vi "Teleop.vi"(6 "Intake speed axis":dbl, 8 "Auto Center":bool, 9 "Outtake":bool, 10 "Intake":bool, 11 "intake.lvclass":refnum<class "intake.lvclass">) -> (2 "State":T1, 3 "intake.lvclass":refnum<class "intake.lvclass">)   [LabVIEW 2015, in "intake.lvclass"]
uses:
  intake.lvclass
  Intake States.ctl
  Robot Global Data.vi
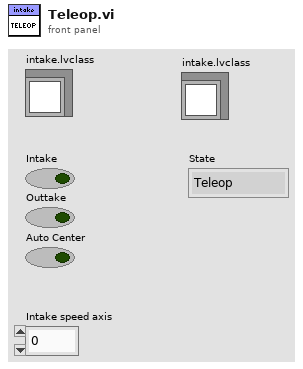
[diagram p1: front panel]
types:
  T1 = typedef "Intake States.ctl" = enum16{"Teleop", "Centering In", "Centering Out"}
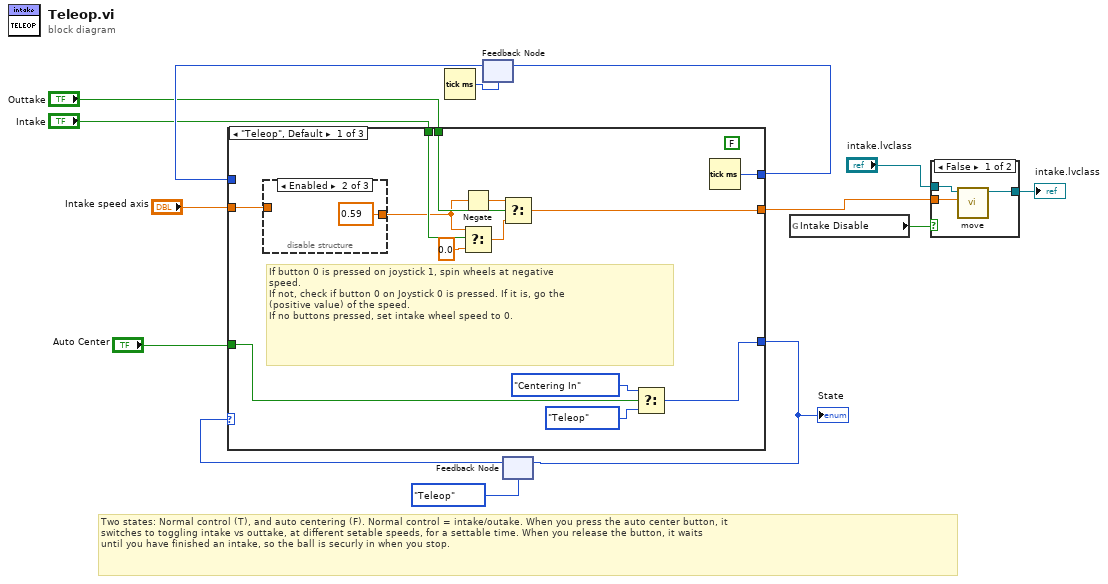
[diagram p0: block diagram]
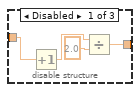
[diagram p2: hidden frame]
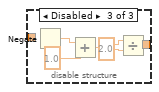
[diagram p3: hidden frame]
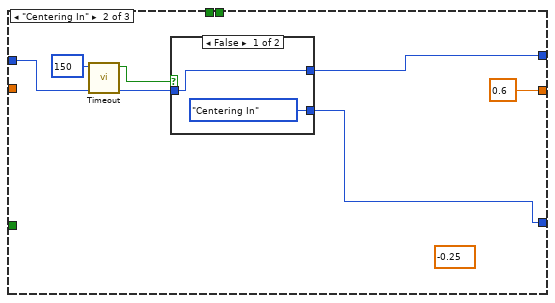
[diagram p4: hidden frame]
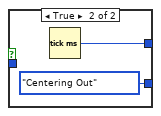
[diagram p5: hidden frame]
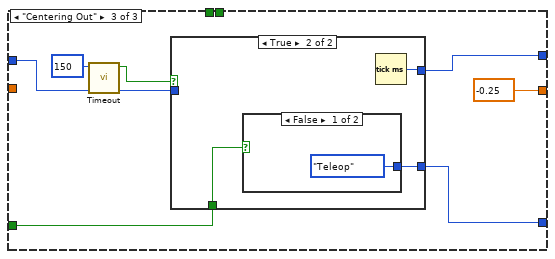
[diagram p6: hidden frame]
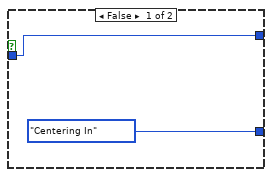
[diagram p7: hidden frame]
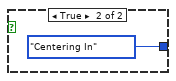
[diagram p8: hidden frame]
diagram:
  # "Two states: Normal control (T), and auto centering (F). Normal control = intake/outake. When you press the auto center button, it \nswitches to toggling intake vs outtake, at different setable speeds, for a settable time. When you release the button, it waits\nuntil you have finished an intake, so the ball is securly in when you stop."
  n1 = Tick Count (ms)() -> (millisecond timer value=w10:u32)
  n2 = feedback #1(w10) -> (w11:u32)
  n3 = feedback #2(Intake_States."Teleop" ("Enum")) -> (w1:T1)
  n4 = case shown="\"Teleop\", Default" w1 {
    tunnel: "Outtake" -> [w25 _ _]
    tunnel: "Intake" -> [w24 _ _]
    tunnel: "Intake speed axis" -> [w22 _ _]
    tunnel: [w20 0.6 ("t") -0.25 ("f")] -> w13
    tunnel: [w19 w41 w53] -> w12
    tunnel: w11 -> [_ w43 w55]
    tunnel: [w15 w38 w51] -> w9
    tunnel: "Auto Center" -> [w18 _ w49]
    frame "Teleop", Default {
      (unwired) FALSE ("Intake Disable")
      # "If button 0 is pressed on joystick 1, spin wheels at negative\nspeed.\nIf not, check if button 0 on Joystick 0 is pressed. If it is, go the\n(positive value) of the speed.\nIf no buttons pressed, set intake wheel speed to 0."
      n5 = disable-structure shown="Enabled" {
        disable-tunnel: w22 -> [w31 _ _]
        disable-tunnel: [w28 0.59 w36] -> w21
        frame Disabled {
          n6 = Increment(x=w31) -> (x+1=w30:dbl)
          n7 = Divide(x=w30, y=2.0) -> (x/y=w28:dbl)
        }
        frame Enabled {
        }
        frame Disabled {
          n8 = Negate() -> (-x=w35:dbl)  [unwired: 1 in]
          n9 = Add(x=w35, y=1.0) -> (x+y=w33:dbl)
          n10 = Divide(x=w33, y=2.0) -> (x/y=w36:dbl)
        }
      }
      n11 = Negate(x=w21) -> (-x=w23:dbl)
      n12 = Select(t=w21, s=w24, f=0.0) -> (s? t:f=w26:dbl)
      n13 = Select(t=w23, s=w25, f=w26) -> (s? t:f=w20:dbl)
      n14 = Select(t=Intake_States."Centering In" ("Enum"), s=w18, f=Intake_States."Teleop" ("Enum")) -> (s? t:f=w15:T1)
      n15 = Tick Count (ms)() -> (millisecond timer value=w19:u32)
    }
    frame "Centering In" {
      (unwired) -0.25 ("f")
      n16 = call "Timeout.vi"("Start Time In"=w43, "Time Limit"=u32 150) -> ("Start Time Out"=w42:u32, "Timeout"=w40:bool)  [unwired: 8 in]
      n17 = case shown="False" w40 {
        tunnel: w42 -> [w46 _]
        tunnel: [w46 w48] -> w41
        tunnel: [Intake_States."Centering In" ("Enum") Intake_States."Centering Out" ("Enum")] -> w38
        frame False {
        }
        frame True {
          n18 = Tick Count (ms)() -> (millisecond timer value=w48:u32)
        }
      }
    }
    frame "Centering Out" {
      n19 = call "Timeout.vi"("Start Time In"=w55, "Time Limit"=u32 150) -> ("Start Time Out"=w54:u32, "Timeout"=w52:bool)  [unwired: 8 in]
      n20 = case shown="True" w52 {
        tunnel: w54 -> [w58 _]
        tunnel: [w58 w60] -> w53
        tunnel: [Intake_States."Centering In" ("Enum") w61] -> w51
        tunnel: w49 -> [_ w59]
        frame False {
        }
        frame True {
          n21 = case shown="False" w59 {
            tunnel: [Intake_States."Teleop" ("Enum") Intake_States."Centering In" ("Enum")] -> w61
            frame False {
            }
            frame True {
            }
          }
          n22 = Tick Count (ms)() -> (millisecond timer value=w60:u32)
        }
      }
    }
  }
  "State" <- w9
  n23 = feedback-in #1(w12) -> ()
  n24 = feedback-in #2(w9) -> ()
  n25 = global read "Robot Global Data.vi" "Intake Disable"() -> (w14:bool)
  n26 = case shown="False" w14 {
    tunnel: w13 -> [w66 _]
    tunnel: "intake.lvclass" -> [w65 w67]
    tunnel: [w64 w67] -> w3
    frame False {
      n27 = call "move.vi"("Speed"=w66, "intake.lvclass"=w65) -> ("intake.lvclass"=w64:refnum<class "intake.lvclass">)  [unwired: 9 in]
    }
    frame True {
    }
  }
  "intake.lvclass" <- w3
